vi "array -- gaussian random.vi"(10 "y":dbl=6.0 format="%#_13g", 11 "Numeric":i32=100) -> (1 "number":dbl=-0.8866647826189812)   [LabVIEW 2021]
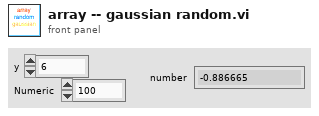
[diagram p1: front panel]
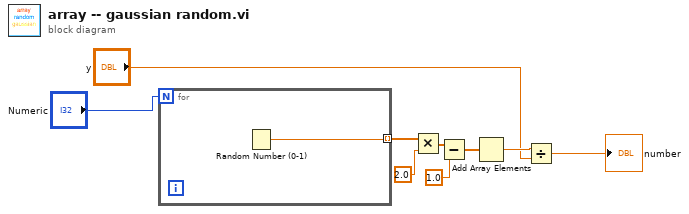
[diagram p0: block diagram]
diagram:
  n1 = for {
    N: "Numeric" -> [_]
    tunnel: [w10] -> w8 mode=indexing
    n2 = Random Number (0-1)() -> (number: 0 to 1=w10:dbl)
  }
  n3 = Multiply(x=w8, y=2.0 ("number (0 to 1)")) -> (x*y=w6:dbl[])
  n4 = Subtract(x=w6, y=1.0 ("number (0 to 1)")) -> (x-y=w4:dbl[])
  n5 = Add Array Elements(numeric array=w4) -> (sum=w3:dbl)
  n6 = Divide(x=w3, y="y") -> (x/y=→"number":dbl)
